vi "extract_shutdown.vi"(5 "multipart message in":string[](array[string]), 11 "error in (no error)":errorcluster) -> (3 "Valid Message?":bool, 14 "Debug info":string, 15 "error out":errorcluster)   [LabVIEW 2019, in "mmW_commands.lvlib"]
uses:
  mmW_commands.lvlib
  TypeDefs/commands.ctl
  typedefs/burst_mode.ctl
  typedefs/instr_hwclass.ctl
  typedefs/mode.ctl
  typedefs/ports.ctl
  Instrument Parameters.ctl
  <vilib>/addons/_JKI.lib/Serialization/JSON/JKI JSON Serialization.lvlib
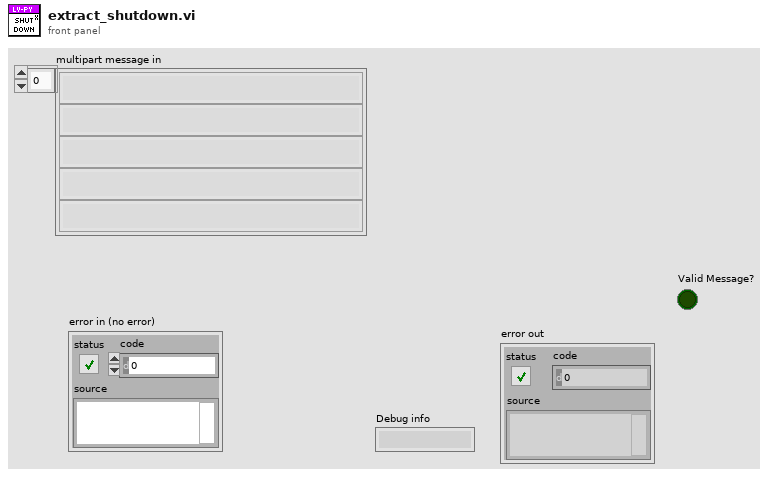
[diagram p1: front panel]
types:
  T1 = typedef "mmW_commands.lvlib/commands.ctl" = enum16{"configure_fs", "configure_rf", "configure_trigger", "equalization_enable", "equalization_start", "lo_sync_enable", "equalization_stop", "get_instrument_status", "get_versions", "initialize_hw", "pop_rx", "set_log_level", "Shutdown", "start", "start_instrument_app", "stop", "trans", "transceive", "trigger_burst", "trigger_sync_enable", "Write TX", "resp_generic", "resp_waveform", "send_trigger", "fetch", "transceive2"}
  T2 = typedef "mmW_commands.lvlib/Instrument Parameters.ctl" = cluster{"Write TX":cluster{"burstname":string, "burst_length":dbl}, "configure_fs":cluster{"port":T3, "fs":dbl}, "configure_rf":cluster{"port":T3, "fc":dbl, "gain":dbl}, "initialize_hw":cluster{"mode":T4, "hwclass":T5}, "start":cluster{"acq_length":dbl, "bursts":string[]}, "trigger_burst":cluster{"burst_mode":T6, "bursts":string[]}, "trigger_sync_enable":cluster{"Enable":bool}, "lo_sync_enable":cluster{"Enable":bool}, "equalization_enable":cluster{"Enable":bool}, "transceive":cluster{"burstname":string, "burst_mode":T6, "bursts":string[], "acq_length":dbl}, "generic_no_param":cluster{"no_param":string}}
  T3 = typedef "mmW_commands.lvlib/ports.ctl" = enum16{"rx", "tx"}
  T4 = typedef "mmW_commands.lvlib/mode.ctl" = enum16{"RF", "IF", "BB"}
  T5 = typedef "mmW_commands.lvlib/instr_hwclass.ctl" = enum16{"Simulated", "NI_mmW01", "Other"}
  T6 = typedef "mmW_commands.lvlib/burst_mode.ctl" = enum16{"burst", "continuous"}
  T7 = enum16{"big-endian, network order", "native, host order", "little-endian"}
  T8 = typedef "mmW_commands.lvlib/datatypes_.ctl" = enum16{"none", "string", "interleaved_I16", "interleaved_I32", "I16_array", "I32_array", "JSONstring"}
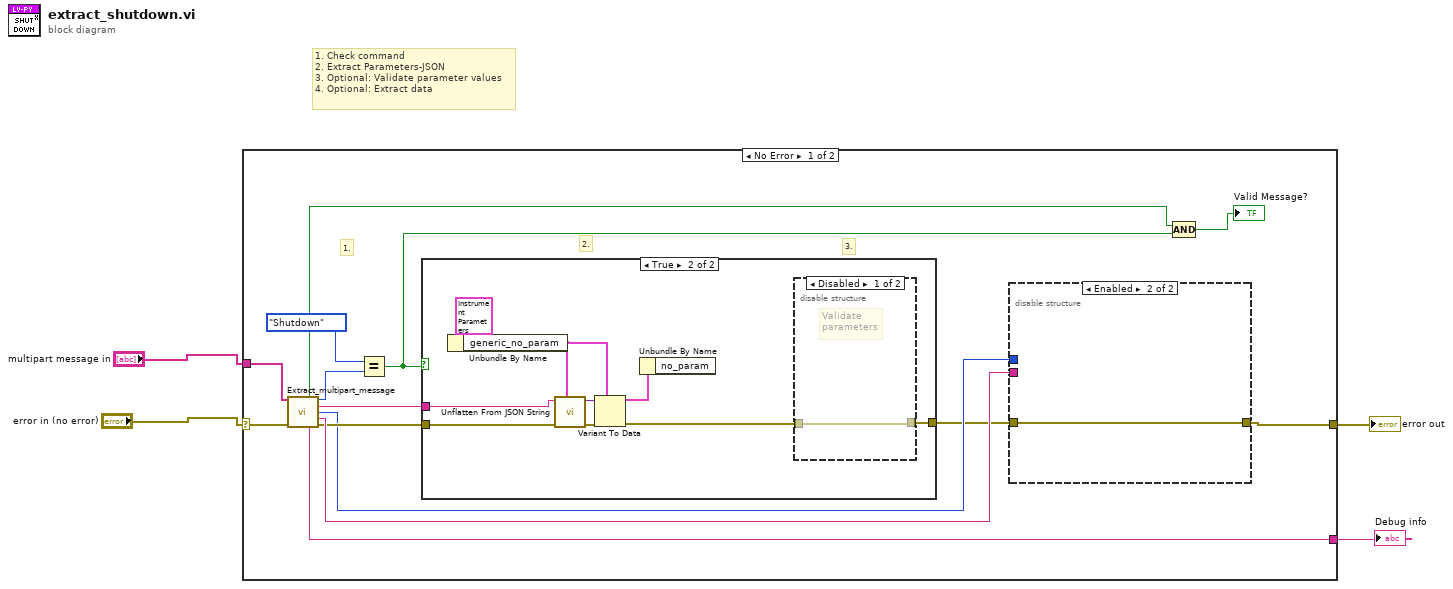
[diagram p0: block diagram]
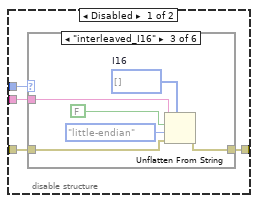
[diagram p4: hidden frame]
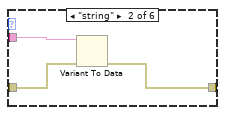
[diagram p6: hidden frame]
diagram:
  # "1. Check command\n2. Extract Parameters-JSON\n3. Optional: Validate parameter values\n4. Optional: Extract data"
  n1 = case shown="No Error" "error in (no error)" {
    selector: "error in (no error)" -> [w18 w48]
    tunnel: [w11 w48] -> w1
    tunnel: "multipart message in" -> [w13 _]
    tunnel: [w17 _] -> w2
    frame No Error {
      # "3."
      # "2."
      # "1."
      n2 = call "Extract_multipart_message.vi"("multipart message in"=w13, "error in (no error)"=w18) -> ("Valid message?"=w8:bool, "command out"=w10:T1, "parameters"=w16:string, "datatype"=w12:T8, "data out"=w15:string, "Debug info"=w17:string, "error out"=w14:errorcluster)  [unwired: 6 in, 1 out]
      n3 = Equal?(x=commands."Shutdown", y=w10) -> (x = y?=w7:bool)
      n4 = case shown="True" w7 {
        tunnel: w16 -> [_ w28]
        tunnel: w14 -> [w19 w25]
        tunnel: [w19 w20] -> w6
        frame False {
        }
        frame True {
          n5 = Unbundle By Name(T2 {"Write TX"={"burstname"="", "burst_length"=0.0}, "configure_fs"={"port"=enum."rx", "fs"=0.0}, "configure_rf"={"port"=enum."rx", "fc"=0.0, "gain"=0.0}, "initialize_hw"={"mode"=enum."RF", "hwclass"=enum."Simulated"}, "start"={"acq_length"=1000.0, "bursts"=[]}, "trigger_burst"={"burst_mode"=enum."burst", "bursts"=[]}, "trigger_sync_enable"={"Enable"=FALSE}, "lo_sync_enable"={"Enable"=FALSE}, "equalization_enable"={"Enable"=FALSE}, "transceive"={"burstname"="", "burst_mode"=enum."burst", "bursts"=[], "acq_length"=1000.0}, "generic_no_param"={"no_param"=""}} ("Instrument parameters")) -> ("generic_no_param"=w23:cluster{"no_param":string})
          n6 = call <vilib>:"Unflatten From JSON String.vi"("Type and Defaults"=w23, "error in (no error)"=w25, "JSON String"=w28) -> ("error out"=w27:errorcluster, "Variant"=w26:variant)  [unwired: 7 in]
          n7 = Variant To Data(error in=w27, type=w23, Variant=w26) -> (data=w22:cluster{"no_param":string}, error out=w21:errorcluster)
          n8 = Unbundle By Name(w22) -> ()  [unwired: 1 out]
          n9 = disable-structure shown="Disabled" {
            disable-tunnel: w21 -> [w29 _]
            disable-tunnel: [w29 _] -> w20
            frame Disabled {
              # "Validate \nparameters"
            }
            frame Enabled {
            }
          }
        }
      }
      n10 = disable-structure shown="Enabled" {
        disable-tunnel: w15 -> [w33 _]
        disable-tunnel: w6 -> [w32 w47]
        disable-tunnel: [w31 w47] -> w11
        disable-tunnel: w12 -> [w30 _]
        frame Disabled {
          n11 = case shown="\"interleaved_I16\"" w30 {
            tunnel: w33 -> [_ w37 w40 _ _ _]
            tunnel: w32 -> [w34 w36 w39 w44 w45 w46]
            tunnel: [w34 w35 w38 w44 w45 w46] -> w31
            frame "none", Default {
            }
            frame "string" {
              n12 = Variant To Data(error in=w36, Variant=w37) -> (error out=w35:errorcluster)  [unwired: 1 in, 1 out]
            }
            frame "interleaved_I16" {
              w43 = i16[] []  # I16
              n13 = Unflatten From String(type=w43, binary string=w40, data includes array or string size? (T)=FALSE, byte order (0:big-endian, network order)=T7."little-endian", error in (no error)=w39) -> (error out=w38:errorcluster)  [unwired: 2 out]
            }
            frame "interleaved_I32" {
            }
            frame "I16_array" {
            }
            frame "I32_array" {
            }
          }
        }
        frame Enabled {
        }
      }
      n14 = Compound Arithmetic op=AND(w8, w7) -> (→"Valid Message?":bool)
    }
    frame Error {
    }
  }
  "error out" <- w1
  "Debug info" <- w2
